vi "bundle DAQmx data for v3.21 .vi"(1 "DAQmx Data":dbl[](array[numeric])) -> (0 "DAQmx Data":T1)   [LabVIEW 2018]
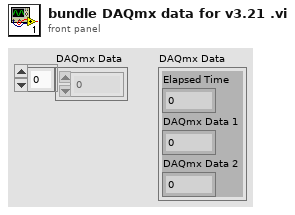
[diagram p1: front panel]
types:
  T1 = cluster{"Elapsed Time":dbl, "DAQmx Data 1":dbl, "DAQmx Data 2":dbl}
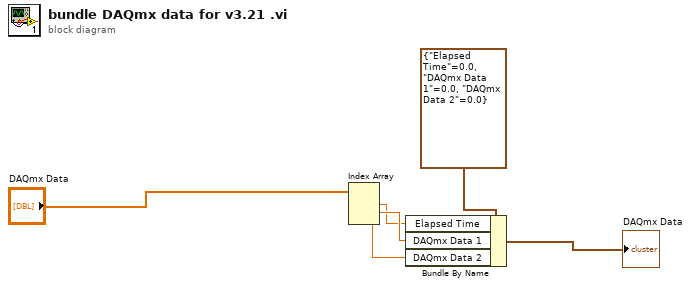
[diagram p0: block diagram]
diagram:
  n1 = Index Array(array="DAQmx Data") -> (element #1=w2:dbl, element #2=w3:dbl, element #3=w5:dbl)  [unwired: 3 in]
  n2 = Bundle By Name(cluster=T1 {"Elapsed Time"=0.0, "DAQmx Data 1"=0.0, "DAQmx Data 2"=0.0}, "Elapsed Time"=w2, "DAQmx Data 1"=w3, "DAQmx Data 2"=w5) -> (→"DAQmx Data":T1)
